vi "Main.vi"() -> ()   [LabVIEW 2019]
uses:
  Etat_Asc.ctl
  Commande 2.ctl
  <vilib>/myRIO/Common/Instrument Driver Framework/myRIO v1.0/DIO/typedefs/DIO Channels Enum.ctl
  <vilib>/myRIO/Common/Instrument Driver Framework/myRIO v1.0/DIO/typedefs/DIO Channels List.ctl
  <vilib>/myRIO/Common/Instrument Driver Framework/Utilities/typedefs/Generic FPGA Reference.ctl
  <vilib>/myRIO/Common/Instrument Driver Framework/Utilities/typedefs/myRIO v1.0 Reference.ctl
  <vilib>/myRIO/Common/Instrument Driver Framework/Utilities/typedefs/Hardware Version Enum.ctl
  <vilib>/myRIO/Common/Instrument Driver Framework/Utilities/typedefs/myRIO Generic Hardware Reference.ctl
  <vilib>/myRIO/Instrument Drivers/Onboard IO/DIO/typedefs/DIO Reference.ctl
  <vilib>/myRIO/Instrument Drivers/Onboard IO/DIO/DIO.lvlib
  <vilib>/userDefined/High Color/nirio_resource_hc.ctl
  <vilib>/myRIO/Common/Instrument Driver Framework/myRIO v1.0/DIO/vis/myRIO v1.1 Open DIO.vi
  <vilib>/myRIO/Instrument Drivers/Onboard IO/DIO/vis/myRIO DIO Open.xnode
  L298N_Ref_Type.ctl
  Asc_State_Inputs.ctl
panel:
  out "error out":errorcluster caption="sortie d'erreur"
  out "Etage_Cible":dbl
  out "Etage_Actuel":dbl
  out "Etat_Actuel":T1
  out "Capteurs_Cabine_Presente":bool[](array[boolean])
  out "Capteurs_Porte_Fermee":bool[](array[boolean])
  out "Capteurs_Porte_Ouverte":bool[](array[boolean])
  in  "stop":bool
  out "Tableau_Appels":bool[](array[boolean])
  in  "Dest_3":bool
  in  "Dest_2":bool
  in  "Dest_1":bool
  in  "Dest_0":bool
  in  "Appel_0":bool
  in  "Appel_3":bool
  in  "Appel_2":bool
  in  "Appel_1":bool
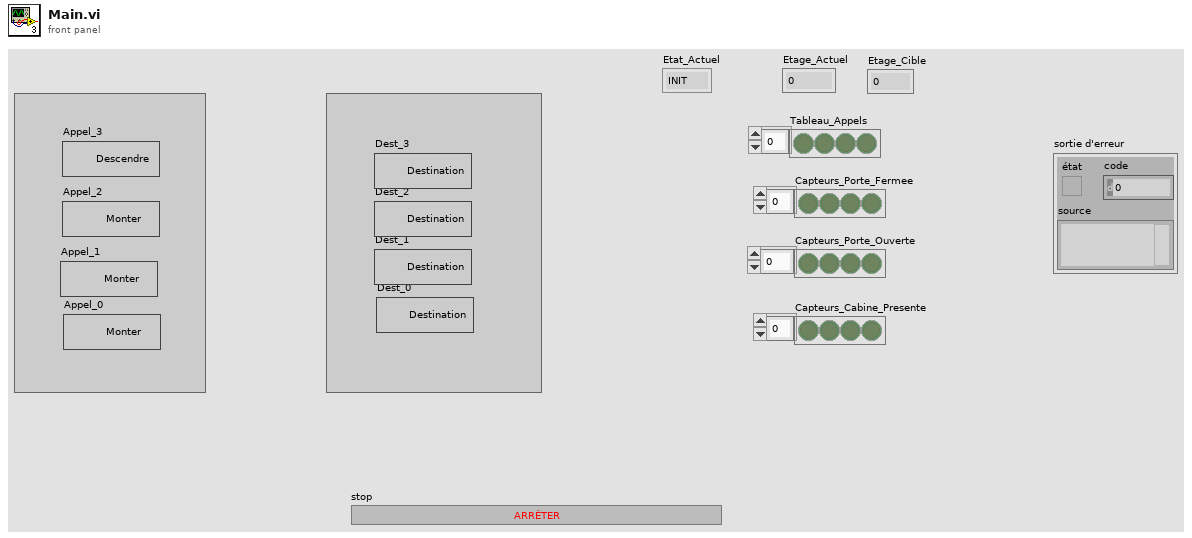
[diagram p1: front panel]
types:
  T1 = typedef "Etat_Asc.ctl" = enum16{"INIT", "REPOS", "DEPLACEMENT", "OUVERTURE_PORTE", "ATTENTE_TEMPO", "FERMETURE_PORTE", "ARRET_URGENCE"}
  T2 = typedef "Commande 2.ctl" = enum16{"INIT", "REPOS", "DEPLACEMENT", "OUVERTURE_PORTE", "ATTENTE_TEMPO", "FERMETURE_PORTE", "ARRET_URGENCE"}
  T3 = typedef "L298N_Ref_Type.ctl" = cluster{"DIO_Ref_Montee":T4, "DIO_Ref_Descente":T4}
  T4 = typedef "DIO.lvlib/DIO Reference.ctl" = cluster{"myRIO Reference":T5, "DIO Channels List":T9}
  T5 = typedef "myRIO Generic Hardware Reference.ctl" = cluster{"myRIO Model":T6, "myRIO Hardware Reference":T7}
  T6 = typedef "Hardware Version Enum.ctl" = enum16{"Unknown", "myRIO-1900", "myRIO-1950", "roboRIO", "NI ELVIS RIO CM", "ELVIS III"}
  T7 = typedef "myRIO v1.0 Reference.ctl" = cluster{"Generic FPGA Reference":T8, "Allow multiple opens":bool}
  T8 = typedef "Generic FPGA Reference.ctl" = refnum<k20>
  T9 = typedef "DIO Channels List.ctl" = T10[]
  T10 = typedef "DIO Channels Enum.ctl" = enum16{"Not Connected", "C/DIO0", "C/DIO1", "C/DIO2", "C/DIO3", "C/DIO4", "C/DIO5", "C/DIO6", "C/DIO7", "A/DIO0", "A/DIO1", "A/DIO2", "A/DIO3", "A/DIO4", "A/DIO5", "A/DIO6", "A/DIO7", "A/DIO8", "A/DIO9", "A/DIO10", "A/DIO11", "A/DIO12", "A/DIO13", "A/DIO14", "A/DIO15", "A/DIO16", "A/DIO17", "A/DIO18", "A/DIO19", "B/DIO0", "B/DIO1", "B/DIO2", "B/DIO3", "B/DIO4", "B/DIO5", "B/DIO6", "B/DIO7", "B/DIO8", "B/DIO9", "B/DIO10", "B/DIO11", "B/DIO12", "B/DIO13", "B/DIO14", "B/DIO15", "B/DIO16", "B/DIO17", "B/DIO18", "B/DIO19", "LED0", "LED1", "LED2", "LED3", "Button0", "DIO/DIO0", "DIO/DIO1", "DIO/DIO2", "DIO/DIO3", "DIO/DIO4", "DIO/DIO5", "DIO/DIO6", "DIO/DIO7", "DIO/DIO8", "DIO/DIO9", "SPI/CS0", "SPI/CS1", "SPI/CS2", "SPI/CS3", "LED RADIO (Green)", "LED RADIO (Red)", "LED COMM (Green)", "LED COMM (Red)", "LED MODE (Green)", "LED MODE (Red)"}
  T11 = typedef "Asc_State_Inputs.ctl" = cluster{"Etage_Actuel":dbl, "Etat_Actuel":T1, "Etage_Cible":dbl, "Tableau_Appels":bool[], "Capteurs_Porte_Ouverte":bool[], "Capteurs_Porte_Fermee":bool[], "Cabine":T3, "Portes":T3[], "Refs_DI_Appels_Couloir":T4[], "Refs_DI_Presence":T4[], "Refs_DI_Porte_Ouverte":T4[], "Refs_DI_Porte_Fermee":T4[], "Capteurs_Cabine_Presente":bool[], "Btn_Appel_Couloir":refnum<vi>[], "Btn_Dest_Cabine":refnum<vi>[]}
  T12 = typedef "nirio_resource_hc.ctl" = tag
  T13 = typedef "Asc_State_Inputs.ctl" = cluster{"Etage_Actuel":i32, "Etat_Actuel":T1, "Etage_Cible":i32, "Tableau_Appels":bool[], "Capteurs_Porte_Ouverte":bool[], "Capteurs_Porte_Fermee":bool[], "Cabine":T3, "Portes":T3[], "Refs_DI_Appels_Couloir":T4[], "Refs_DI_Presence":T4[], "Refs_DI_Porte_Ouverte":T4[], "Refs_DI_Porte_Fermee":T4[], "Capteurs_Cabine_Presente":bool[], "Btn_Appel_Couloir":refnum<vi>[], "Btn_Dest_Cabine":refnum<vi>[]}
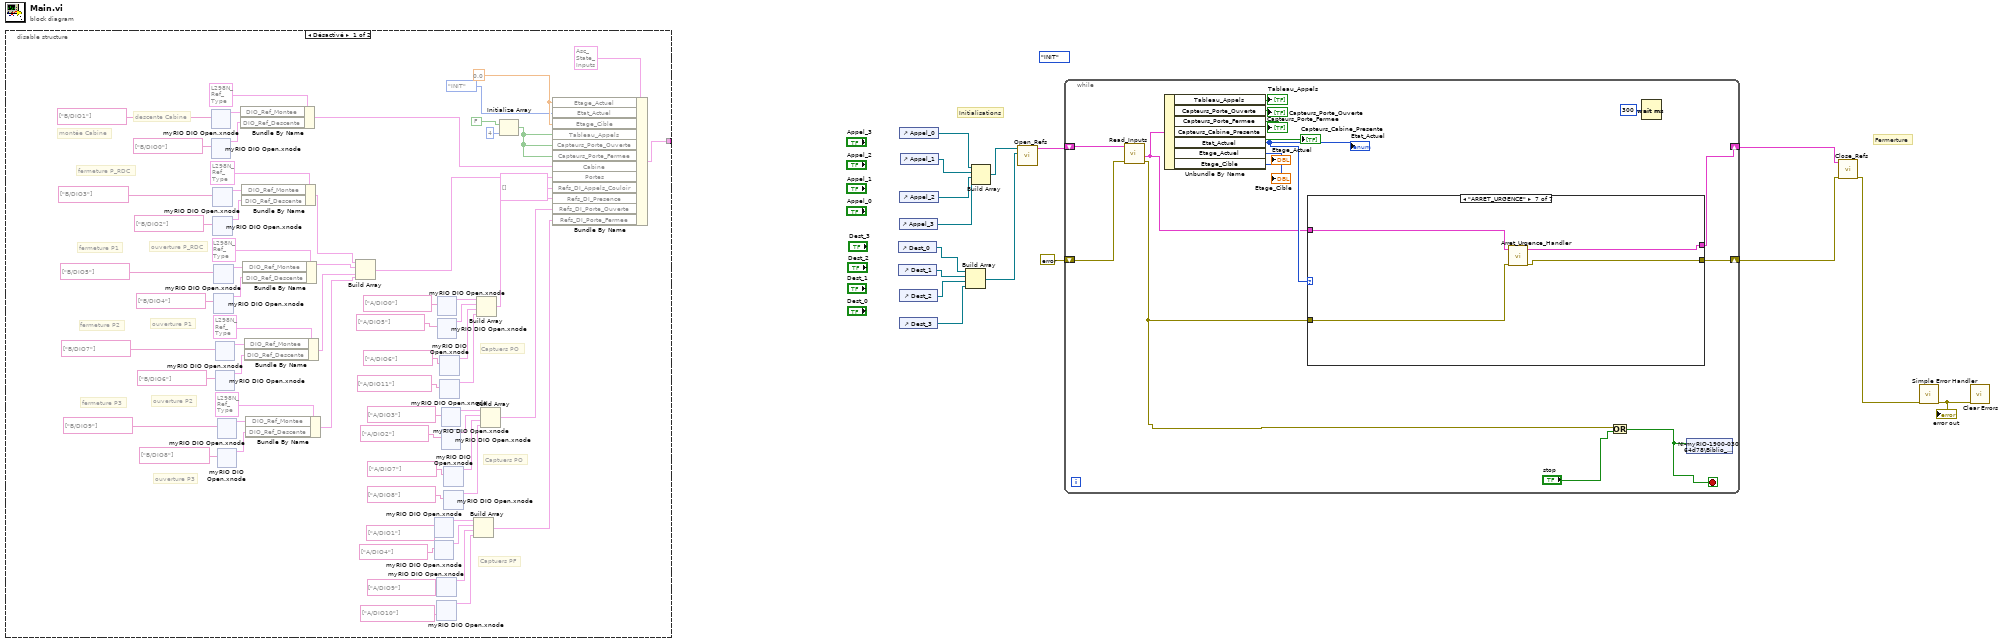
[diagram p0: block diagram]
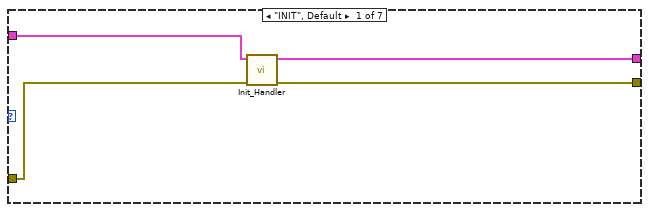
[diagram p3: hidden frame]
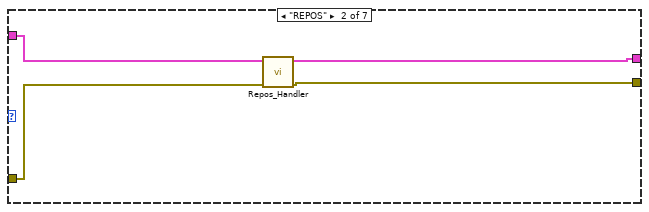
[diagram p4: hidden frame]
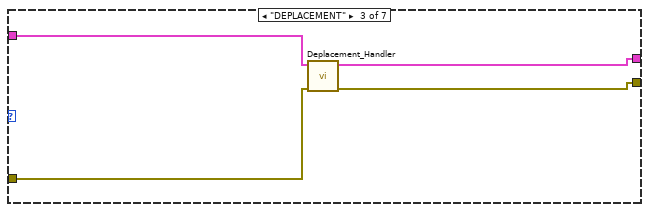
[diagram p5: hidden frame]
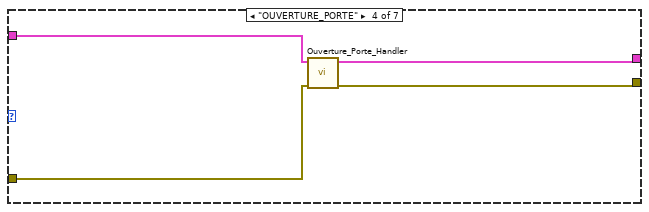
[diagram p6: hidden frame]
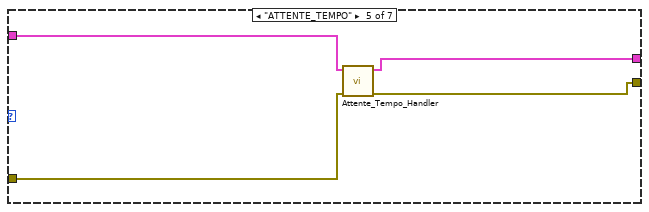
[diagram p7: hidden frame]
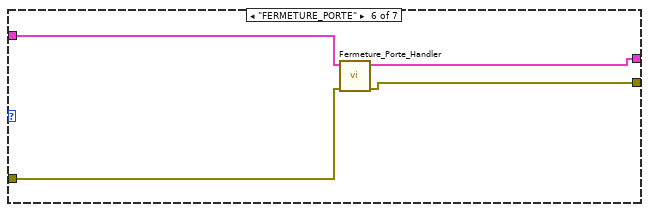
[diagram p8: hidden frame]
diagram:
  (unwired) Commande_2."INIT" ("Etat_Asc")
  # "Fermerture"
  # "Initialisations"
  n1 = disable-structure shown="Désactivé" {
    disable-tunnel: [w55 _] -> _
    frame Disabled {
      w54 = 0.0 ("Etage_Actuel")
      # "montée Cabine"
      # "descente Cabine"
      # "Captuers PO"
      # "Captuers PO"
      # "Captuers PF"
      # "fermeture P3"
      # "ouverture P3"
      # "fermeture P2"
      # "ouverture P2"
      # "fermeture P1"
      # "ouverture P1"
      # "fermeture P_RDC"
      # "ouverture P_RDC"
      n2 = xnode "myRIO DIO Open.xnode"("Channel Names"=tag[] ["B/DIO1"]) -> ("DIO Ref Out"=w19:T4)  [unwired: 2 in, 1 out]
      n3 = xnode "myRIO DIO Open.xnode"("Channel Names"=tag[] ["B/DIO0"]) -> ("DIO Ref Out"=w18:T4)  [unwired: 2 in, 1 out]
      n4 = xnode "myRIO DIO Open.xnode"("Channel Names"=tag[] ["B/DIO3"]) -> ("DIO Ref Out"=w80:T4)  [unwired: 2 in, 1 out]
      n5 = xnode "myRIO DIO Open.xnode"("Channel Names"=tag[] ["B/DIO2"]) -> ("DIO Ref Out"=w81:T4)  [unwired: 2 in, 1 out]
      n6 = xnode "myRIO DIO Open.xnode"("Channel Names"=tag[] ["B/DIO5"]) -> ("DIO Ref Out"=w75:T4)  [unwired: 2 in, 1 out]
      n7 = xnode "myRIO DIO Open.xnode"("Channel Names"=tag[] ["B/DIO4"]) -> ("DIO Ref Out"=w74:T4)  [unwired: 2 in, 1 out]
      n8 = xnode "myRIO DIO Open.xnode"("Channel Names"=tag[] ["B/DIO7"]) -> ("DIO Ref Out"=w70:T4)  [unwired: 2 in, 1 out]
      n9 = xnode "myRIO DIO Open.xnode"("Channel Names"=tag[] ["B/DIO6"]) -> ("DIO Ref Out"=w71:T4)  [unwired: 2 in, 1 out]
      n10 = xnode "myRIO DIO Open.xnode"("Channel Names"=tag[] ["B/DIO9"]) -> ("DIO Ref Out"=w65:T4)  [unwired: 2 in, 1 out]
      n11 = xnode "myRIO DIO Open.xnode"("Channel Names"=tag[] ["B/DIO8"]) -> ("DIO Ref Out"=w64:T4)  [unwired: 2 in, 1 out]
      n12 = Bundle By Name(cluster=T3 {"DIO_Ref_Montee"={"myRIO Reference"={"myRIO Model"=enum."Unknown", "myRIO Hardware Reference"={"Generic FPGA Reference"=refnum, "Allow multiple opens"=FALSE}}, "DIO Channels List"=[]}, "DIO_Ref_Descente"={"myRIO Reference"={"myRIO Model"=enum."Unknown", "myRIO Hardware Reference"={"Generic FPGA Reference"=refnum, "Allow multiple opens"=FALSE}}, "DIO Channels List"=[]}} ("Cluster 2"), "DIO_Ref_Montee"=w19, "DIO_Ref_Descente"=w18) -> (w57:T3)
      n13 = Bundle By Name(cluster=T3 {"DIO_Ref_Montee"={"myRIO Reference"={"myRIO Model"=enum."Unknown", "myRIO Hardware Reference"={"Generic FPGA Reference"=refnum, "Allow multiple opens"=FALSE}}, "DIO Channels List"=[]}, "DIO_Ref_Descente"={"myRIO Reference"={"myRIO Model"=enum."Unknown", "myRIO Hardware Reference"={"Generic FPGA Reference"=refnum, "Allow multiple opens"=FALSE}}, "DIO Channels List"=[]}} ("Cluster 2"), "DIO_Ref_Montee"=w80, "DIO_Ref_Descente"=w81) -> (w62:T3)
      n14 = Bundle By Name(cluster=T3 {"DIO_Ref_Montee"={"myRIO Reference"={"myRIO Model"=enum."Unknown", "myRIO Hardware Reference"={"Generic FPGA Reference"=refnum, "Allow multiple opens"=FALSE}}, "DIO Channels List"=[]}, "DIO_Ref_Descente"={"myRIO Reference"={"myRIO Model"=enum."Unknown", "myRIO Hardware Reference"={"Generic FPGA Reference"=refnum, "Allow multiple opens"=FALSE}}, "DIO Channels List"=[]}} ("Cluster 2"), "DIO_Ref_Montee"=w75, "DIO_Ref_Descente"=w74) -> (w61:T3)
      n15 = Bundle By Name(cluster=T3 {"DIO_Ref_Montee"={"myRIO Reference"={"myRIO Model"=enum."Unknown", "myRIO Hardware Reference"={"Generic FPGA Reference"=refnum, "Allow multiple opens"=FALSE}}, "DIO Channels List"=[]}, "DIO_Ref_Descente"={"myRIO Reference"={"myRIO Model"=enum."Unknown", "myRIO Hardware Reference"={"Generic FPGA Reference"=refnum, "Allow multiple opens"=FALSE}}, "DIO Channels List"=[]}} ("Cluster 2"), "DIO_Ref_Montee"=w70, "DIO_Ref_Descente"=w71) -> (w60:T3)
      n16 = Bundle By Name(cluster=T3 {"DIO_Ref_Montee"={"myRIO Reference"={"myRIO Model"=enum."Unknown", "myRIO Hardware Reference"={"Generic FPGA Reference"=refnum, "Allow multiple opens"=FALSE}}, "DIO Channels List"=[]}, "DIO_Ref_Descente"={"myRIO Reference"={"myRIO Model"=enum."Unknown", "myRIO Hardware Reference"={"Generic FPGA Reference"=refnum, "Allow multiple opens"=FALSE}}, "DIO Channels List"=[]}} ("Cluster 2"), "DIO_Ref_Montee"=w65, "DIO_Ref_Descente"=w64) -> (w59:T3)
      n17 = Build Array(w62, w61, w60, w59) -> (w56:T3[])
      n18 = xnode "myRIO DIO Open.xnode"("Channel Names"=tag[] ["A/DIO1"]) -> ("DIO Ref Out"=w34:T4)  [unwired: 2 in, 1 out]
      n19 = xnode "myRIO DIO Open.xnode"("Channel Names"=tag[] ["A/DIO4"]) -> ("DIO Ref Out"=w37:T4)  [unwired: 2 in, 1 out]
      n20 = xnode "myRIO DIO Open.xnode"("Channel Names"=tag[] ["A/DIO9"]) -> ("DIO Ref Out"=w36:T4)  [unwired: 2 in, 1 out]
      n21 = xnode "myRIO DIO Open.xnode"("Channel Names"=tag[] ["A/DIO10"]) -> ("DIO Ref Out"=w35:T4)  [unwired: 2 in, 1 out]
      n22 = xnode "myRIO DIO Open.xnode"("Channel Names"=tag[] ["A/DIO0"]) -> ("DIO Ref Out"=w31:T4)  [unwired: 2 in, 1 out]
      n23 = xnode "myRIO DIO Open.xnode"("Channel Names"=tag[] ["A/DIO5"]) -> ("DIO Ref Out"=w28:T4)  [unwired: 2 in, 1 out]
      n24 = xnode "myRIO DIO Open.xnode"("Channel Names"=tag[] ["A/DIO6"]) -> ("DIO Ref Out"=w29:T4)  [unwired: 2 in, 1 out]
      n25 = xnode "myRIO DIO Open.xnode"("Channel Names"=tag[] ["A/DIO11"]) -> ("DIO Ref Out"=w30:T4)  [unwired: 2 in, 1 out]
      n26 = xnode "myRIO DIO Open.xnode"("Channel Names"=tag[] ["A/DIO3"]) -> ("DIO Ref Out"=w49:T4)  [unwired: 2 in, 1 out]
      n27 = xnode "myRIO DIO Open.xnode"("Channel Names"=tag[] ["A/DIO2"]) -> ("DIO Ref Out"=w46:T4)  [unwired: 2 in, 1 out]
      n28 = xnode "myRIO DIO Open.xnode"("Channel Names"=tag[] ["A/DIO7"]) -> ("DIO Ref Out"=w47:T4)  [unwired: 2 in, 1 out]
      n29 = xnode "myRIO DIO Open.xnode"("Channel Names"=tag[] ["A/DIO8"]) -> ("DIO Ref Out"=w48:T4)  [unwired: 2 in, 1 out]
      n30 = Build Array(w34, w37, w36, w35) -> (w33:T4[])
      n31 = Build Array(w31, w28, w29, w30) -> (w23:T4[])
      n32 = Build Array(w49, w46, w47, w48) -> (w32:T4[])
      n33 = Initialize Array(FALSE, 4 ("taille de la dimension")) -> (w50:bool[])
      n34 = Bundle By Name(cluster=T11 {"Etage_Actuel"=0.0, "Etat_Actuel"=enum."INIT", "Etage_Cible"=0.0, "Tableau_Appels"=[], "Capteurs_Porte_Ouverte"=[], "Capteurs_Porte_Fermee"=[], "Cabine"={"DIO_Ref_Montee"={"myRIO Reference"={"myRIO Model"=enum."Unknown", "myRIO Hardware Reference"={"Generic FPGA Reference"=refnum, "Allow multiple opens"=FALSE}}, "DIO Channels List"=[]}, "DIO_Ref_Descente"={"myRIO Reference"={"myRIO Model"=enum."Unknown", "myRIO Hardware Reference"={"Generic FPGA Reference"=refnum, "Allow multiple opens"=FALSE}}, "DIO Channels List"=[]}}, "Portes"=[], "Refs_DI_Appels_Couloir"=[], "Refs_DI_Presence"=[], "Refs_DI_Porte_Ouverte"=[], "Refs_DI_Porte_Fermee"=[], "Capteurs_Cabine_Presente"=[], "Btn_Appel_Couloir"=[], "Btn_Dest_Cabine"=[]} ("State_Params"), "Etage_Actuel"=w54, "Etat_Actuel"=Etat_Asc."INIT", "Etage_Cible"=w54, "Tableau_Appels"=w50, "Capteurs_Porte_Ouverte"=w50, "Capteurs_Porte_Fermee"=w50, "Cabine"=w57, "Portes"=w56, "Refs_DI_Appels_Couloir"=T4[] [], "Refs_DI_Presence"=w23, "Refs_DI_Porte_Ouverte"=w32, "Refs_DI_Porte_Fermee"=w33) -> (w55:T11)
    }
    frame Enabled {
    }
  }
  n35 = control-ref of="Dest_0"() -> (w5:refnum<vi>)
  n36 = control-ref of="Dest_1"() -> (w6:refnum<vi>)
  n37 = control-ref of="Appel_3"() -> (w8:refnum<vi>)
  n38 = control-ref of="Dest_2"() -> (w3:refnum<vi>)
  n39 = control-ref of="Dest_3"() -> (w4:refnum<vi>)
  n40 = control-ref of="Appel_0"() -> (w10:refnum<vi>)
  n41 = control-ref of="Appel_2"() -> (w7:refnum<vi>)
  n42 = control-ref of="Appel_1"() -> (w9:refnum<vi>)
  n43 = Build Array(w5, w6, w3, w4) -> (w2:refnum<vi>[])
  n44 = Build Array(w10, w9, w7, w8) -> (w1:refnum<vi>[])
  n45 = call "Open_Refs.vi"("Refs_Destination_Cabine"=w2, "Ref_Appel_Couloir"=w1) -> ("Donnees_Globale_Out"=w11:T13)  [unwired: 9 in]
  n46 = while {
    shift-right: [w438] -> w15
    shift-left: w11 -> [w450]
    shift-right: [w437] -> w13
    shift-left: errorcluster {"status"=FALSE, "code"=0, "source"=""} ("Error Out") -> [w436]
    stop <- w435 stop-if-true
    n47 = call "Read_Inputs.vi"("Error In"=w436, "Donnees_Globales_IN"=w450) -> ("Error Out"=w440:errorcluster, "Donnees_Globale_Out"=w439:T13)  [unwired: 8 in]
    n48 = Unbundle By Name(w439) -> ("Tableau_Appels"=→"Tableau_Appels":bool[], "Capteurs_Porte_Ouverte"=→"Capteurs_Porte_Ouverte":bool[], "Capteurs_Porte_Fermee"=→"Capteurs_Porte_Fermee":bool[], "Capteurs_Cabine_Presente"=→"Capteurs_Cabine_Presente":bool[], "Etat_Actuel"=w441:T1, "Etage_Actuel"=→"Etage_Actuel":i32, "Etage_Cible"=→"Etage_Cible":i32)
    "Etat_Actuel" <- w441
    n49 = case shown="\"ARRET_URGENCE\"" w441 {
      tunnel: w439 -> [w454 w458 w460 w464 w467 w471 w476]
      tunnel: w440 -> [w453 w457 w459 w463 w468 w472 w475]
      tunnel: [w452 w456 w462 w466 w470 w474 w477] -> w438
      tunnel: [w451 w455 w461 w465 w469 w473 w478] -> w437
      frame "INIT", Default {
        n50 = call "Init_Handler.vi"("Error In"=w453, "Donnees_Globales_IN"=w454) -> ("Error Out"=w451:errorcluster, "Donnees_Globale_Out"=w452:T13)  [unwired: 8 in]
      }
      frame "REPOS" {
        n51 = call "Repos_Handler.vi"("Error In"=w457, "Donnees_Globales_IN"=w458) -> ("Error Out"=w455:errorcluster, "Donnees_Globale_Out"=w456:T13)  [unwired: 8 in]
      }
      frame "DEPLACEMENT" {
        n52 = call "Deplacement_Handler.vi"("Error In"=w459, "Donnees_Globales_IN"=w460) -> ("Error Out"=w461:errorcluster, "Donnees_Globale_Out"=w462:T13)  [unwired: 8 in]
      }
      frame "OUVERTURE_PORTE" {
        n53 = call "Ouverture_Porte_Handler.vi"("Error In"=w463, "Donnees_Globales_IN"=w464) -> ("Error Out"=w465:errorcluster, "Donnees_Globale_Out"=w466:T13)  [unwired: 8 in]
      }
      frame "ATTENTE_TEMPO" {
        n54 = call "Attente_Tempo_Handler.vi"("Error In"=w468, "Donnees_Globales_IN"=w467) -> ("Error Out"=w469:errorcluster, "Donnees_Globale_Out"=w470:T13)  [unwired: 8 in]
      }
      frame "FERMETURE_PORTE" {
        n55 = call "Fermeture_Porte_Handler.vi"("Error In"=w472, "Donnees_Globales_IN"=w471) -> ("Error Out"=w473:errorcluster, "Donnees_Globale_Out"=w474:T13)  [unwired: 8 in]
      }
      frame "ARRET_URGENCE" {
        n56 = call "Arret_Urgence_Handler.vi"("Error In"=w475, "Donnees_Globales_IN"=w476) -> ("Error Out"=w478:errorcluster, "Donnees_Globale_Out"=w477:T13)  [unwired: 8 in]
      }
    }
    n57 = Or(x=w440, y="stop") -> (x .or. y?=w435:bool)
    n58 = Wait (ms)(milliseconds to wait=u32 300 ("attente (ms)")) -> ()  [unwired: 1 out]
    n59 = shared-variable "NI-myRIO-1900-03064d78\\Biblio_Shared_Var.lvlib\\STOP"(w435) -> ()  [unwired: 1 in, 1 out]
  }
  n60 = call "Close_Refs.vi"("Error In"=w13, "Donnees_Globales_IN"=w15) -> ("Error Out"=w14:errorcluster)  [unwired: 9 in]
  n61 = call <vilib>:"Simple Error Handler.vi"("error in (no error)"=w14) -> ("error out"=w16:errorcluster)  [unwired: 4 in, 4 out]
  "error out" <- w16
  n62 = call <vilib>:"Clear Errors.vi"("error in (no error)"=w16) -> ()  [unwired: 5 in, 2 out]
